vi "CPP-8116MetAttach.vi"() -> ()   [LabVIEW 2016]
uses:
  Globals/Meas_global.vi
panel:
  out "Plug in titles":string[](array[string])
  out "Plug in values":string[](array[string])
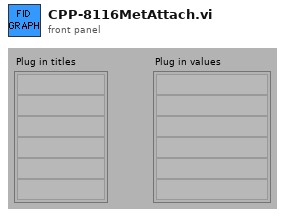
[diagram p1: front panel]
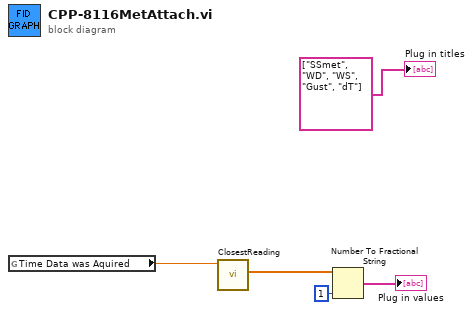
[diagram p0: block diagram]
diagram:
  n1 = global read "Meas_global.vi" "Time Data was Aquired"() -> (w4:dbl)
  n2 = call "ClosestReading.vi"("SS"=w4) -> ("ClosestRow"=w3:dbl[])  [unwired: 10 in]
  n3 = Number To Fractional String(number=w3, precision (6)=i16 1) -> (F-format string=→"Plug in values":string[])  [unwired: 2 in]
  "Plug in titles" <- string[] ["SSmet", "WD", "WS", "Gust", "dT"] ("Plug in titles")
